vi "4.vi"() -> ()   [LabVIEW 2020]
panel:
  in  "STOP":bool
  out "Time Elapsed [ms]":u32
  in  "Action":enum16{"Reset", "Run", "Pause"}(ring)
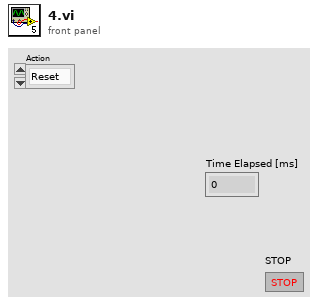
[diagram p1: front panel]
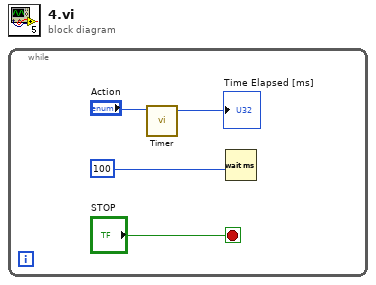
[diagram p0: block diagram]
diagram:
  n1 = while {
    stop <- "STOP" stop-if-true
    n2 = call "Timer.vi"("Action"="Action") -> ("Time Elapsed [ms]"=→"Time Elapsed [ms]":u32)  [unwired: 9 in, 1 out]
    n3 = Wait (ms)(milliseconds to wait=u32 100) -> ()  [unwired: 1 out]
  }
